vi "HTML_BUILDER.vi"(8 "Error In":errorcluster, 10 "Body":cluster{"Description":string, "Path":path}[](array[cluster]), 11 "Head":cluster{"Title":string, "Created":string}) -> (0 "Error Out":errorcluster, 3 "HTML request":T1(array[cluster]))   [LabVIEW 2016]
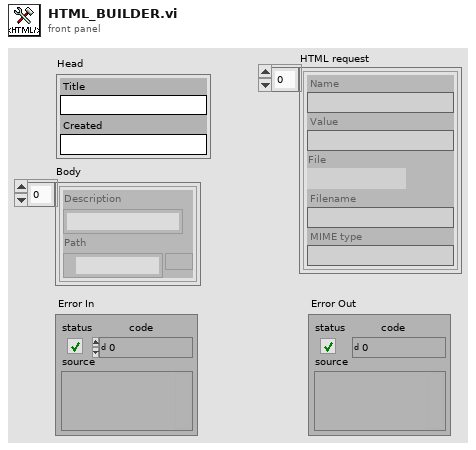
[diagram p1: front panel]
types:
  T1 = cluster{"Name":string, "Value":string, "File":path, "Filename":string, "MIME type":string}[]
  T2 = cluster{"Name":string, "Value":string, "File":path, "Filename":string, "MIME type":string}
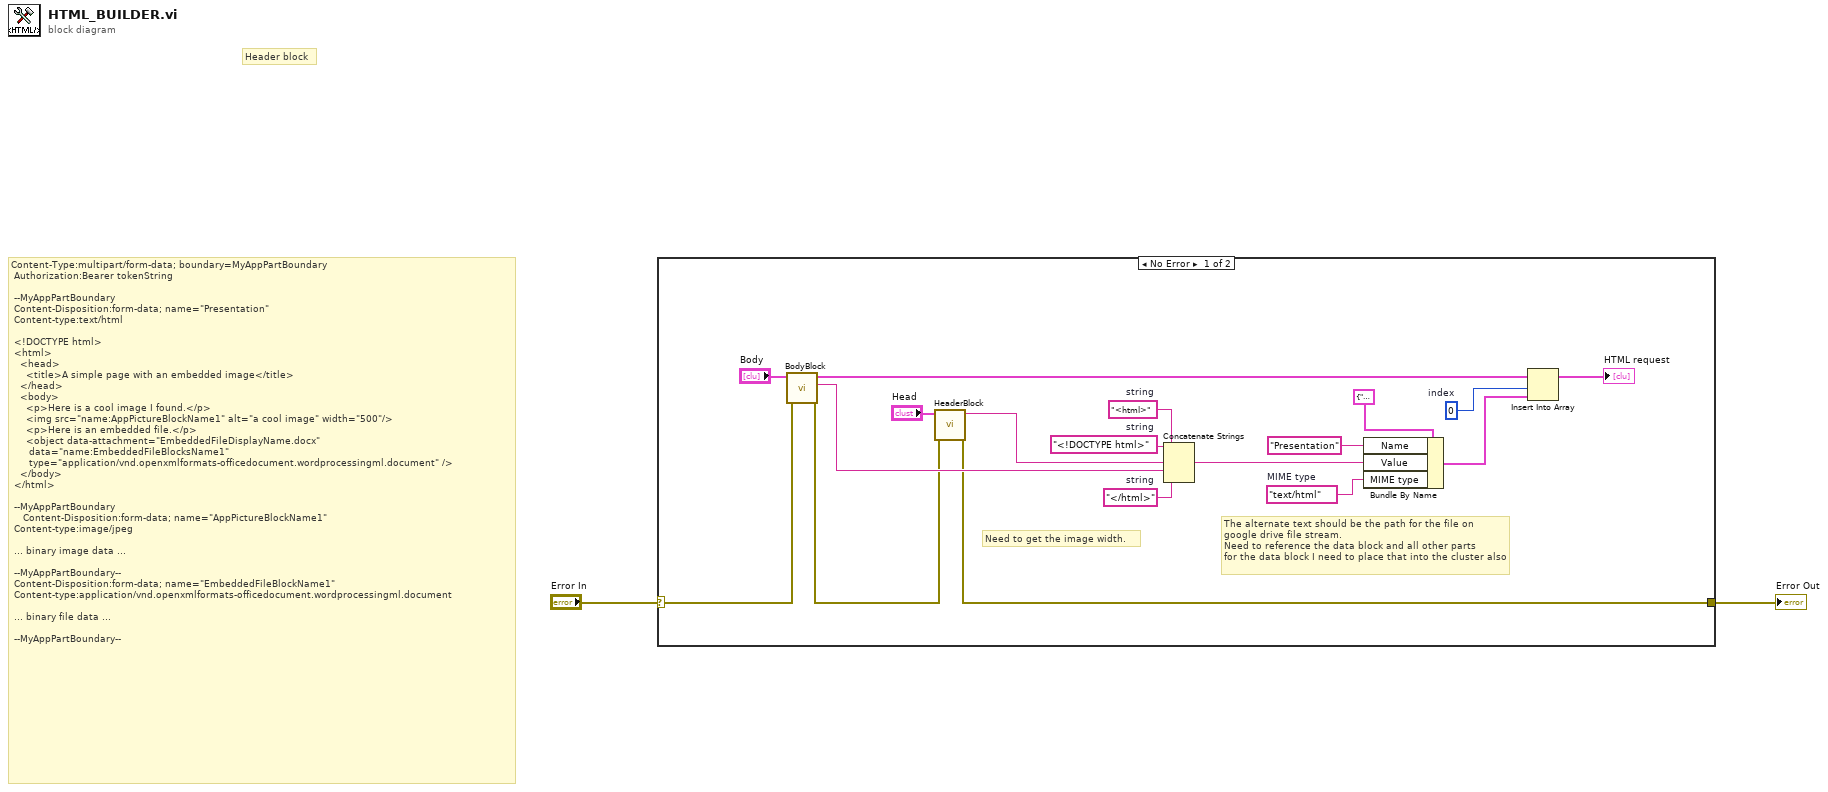
[diagram p0: block diagram]
diagram:
  # "Content-Type:multipart/form-data; boundary=MyAppPartBoundary \n Authorization:Bearer tokenString \n\n --MyAppPartBoundary \n Content-Disposition:form-data; name=\"Presentation\" \n Content-type:text/html \n\n <!DOCTYPE html> \n <html> \n   <head> \n     <title>A simple page with an embedded image</title> \n   </head> \n   <body> \n     <p>Here is a cool image I found.</p> \n     <img src=\"name:AppPictureBlockName1\" alt=\"a cool image\" width=\"500\"/> \n     <p>Here is an embedded file.</p> \n     <object data-attachment=\"EmbeddedFileDisplayName.docx\" \n      data=\"name:EmbeddedFileBlocksName1\" \n      type=\"application/vnd.openxmlformats-officedocument.wordprocessingml.document\" /> \n   </body> \n </html> \n\n --MyAppPartBoundary \n    Content-Disposition:form-data; name=\"AppPictureBlockName1\" \n Content-type:image/jpeg \n\n ... binary image data ... \n\n --MyAppPartBoundary-- \n Content-Disposition:form-data; name=\"EmbeddedFileBlockName1\" \n Content-type:application/vnd.openxmlformats-officedocument.wordprocessingml.document \n\n ... binary file data ... \n\n --MyAppPartBoundary--"
  # "Header block"
  n1 = case shown="No Error" "Error In" {
    selector: "Error In" -> [w3 w21]
    tunnel: [w4 w21] -> w1
    frame No Error {
      w6 = "</html>"  # string
      w7 = "<html>"  # string
      w8 = "<!DOCTYPE html>"  # string
      w12 = 0  # index
      w17 = "text/html"  # MIME type
      # "Need to get the image width."
      # "The alternate text should be the path for the file on google drive file stream.\nNeed to reference the data block and all other parts\nfor the data block I need to place that into the cluster also"
      n2 = call "BodyBlock.vi"("error in (no error)"=w3, "Body"="Body") -> ("error out"=w5:errorcluster, "Body Out"=w9:string, "File Blocks Out"=w13:T1)  [unwired: 6 in]
      n3 = call "HeaderBlock.vi"("error in (no error)"=w5, "Head"="Head") -> ("error out"=w4:errorcluster, "Header Block Out"=w18:string)  [unwired: 8 in]
      n4 = Concatenate Strings(w8, w7, w18, w9, w6) -> (w10:string)
      n5 = Bundle By Name(cluster=T2 {"Name"="", "Value"="", "File"=path "", "Filename"="", "MIME type"="application/octet-stream"} ("Element"), "Name"="Presentation", "Value"=w10, "MIME type"=w17) -> (w14:T2)
      n6 = Insert Into Array(array=w13, index=w12, new element=w14) -> (→"HTML request":T1)
    }
    frame Error {
    }
  }
  "Error Out" <- w1
